vi "Deserialize Object UPDT (XML).vi"(8 "error in":errorcluster, 9 "values":string[](array[string]), 10 "names":string[](array[string]), 11 "object type":refnum<class "_ISerializable.lvclass">) -> (0 "error out":errorcluster, 3 "object out":refnum<class "_ISerializable.lvclass">)   [LabVIEW 2018, in "Serializer.lvclass"]
uses:
  Serializer.lvclass
  _Serializable Base Object/_ISerializable.lvclass
  <vilib>/xml/Close Reference(Node).vi
  <resource>/objmgr/DOMUserDefRef.rc
  <vilib>/xml/NI_XML.lvlib
panel:
  out "XML":string
  out "object xml string":string
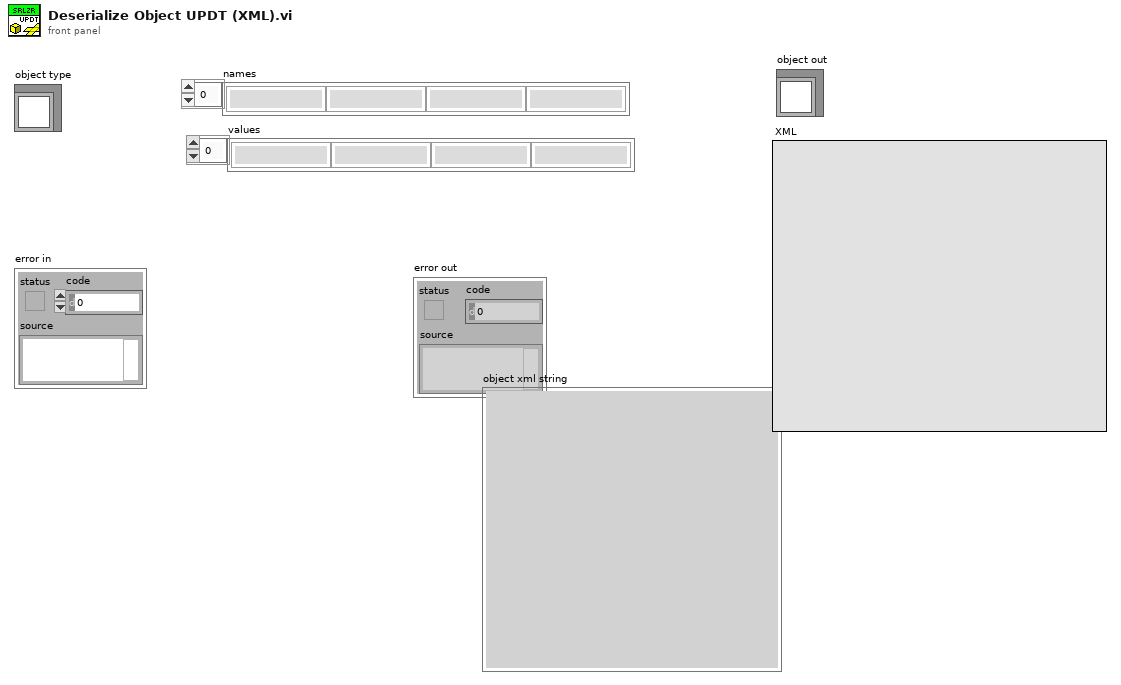
[diagram p1: front panel]
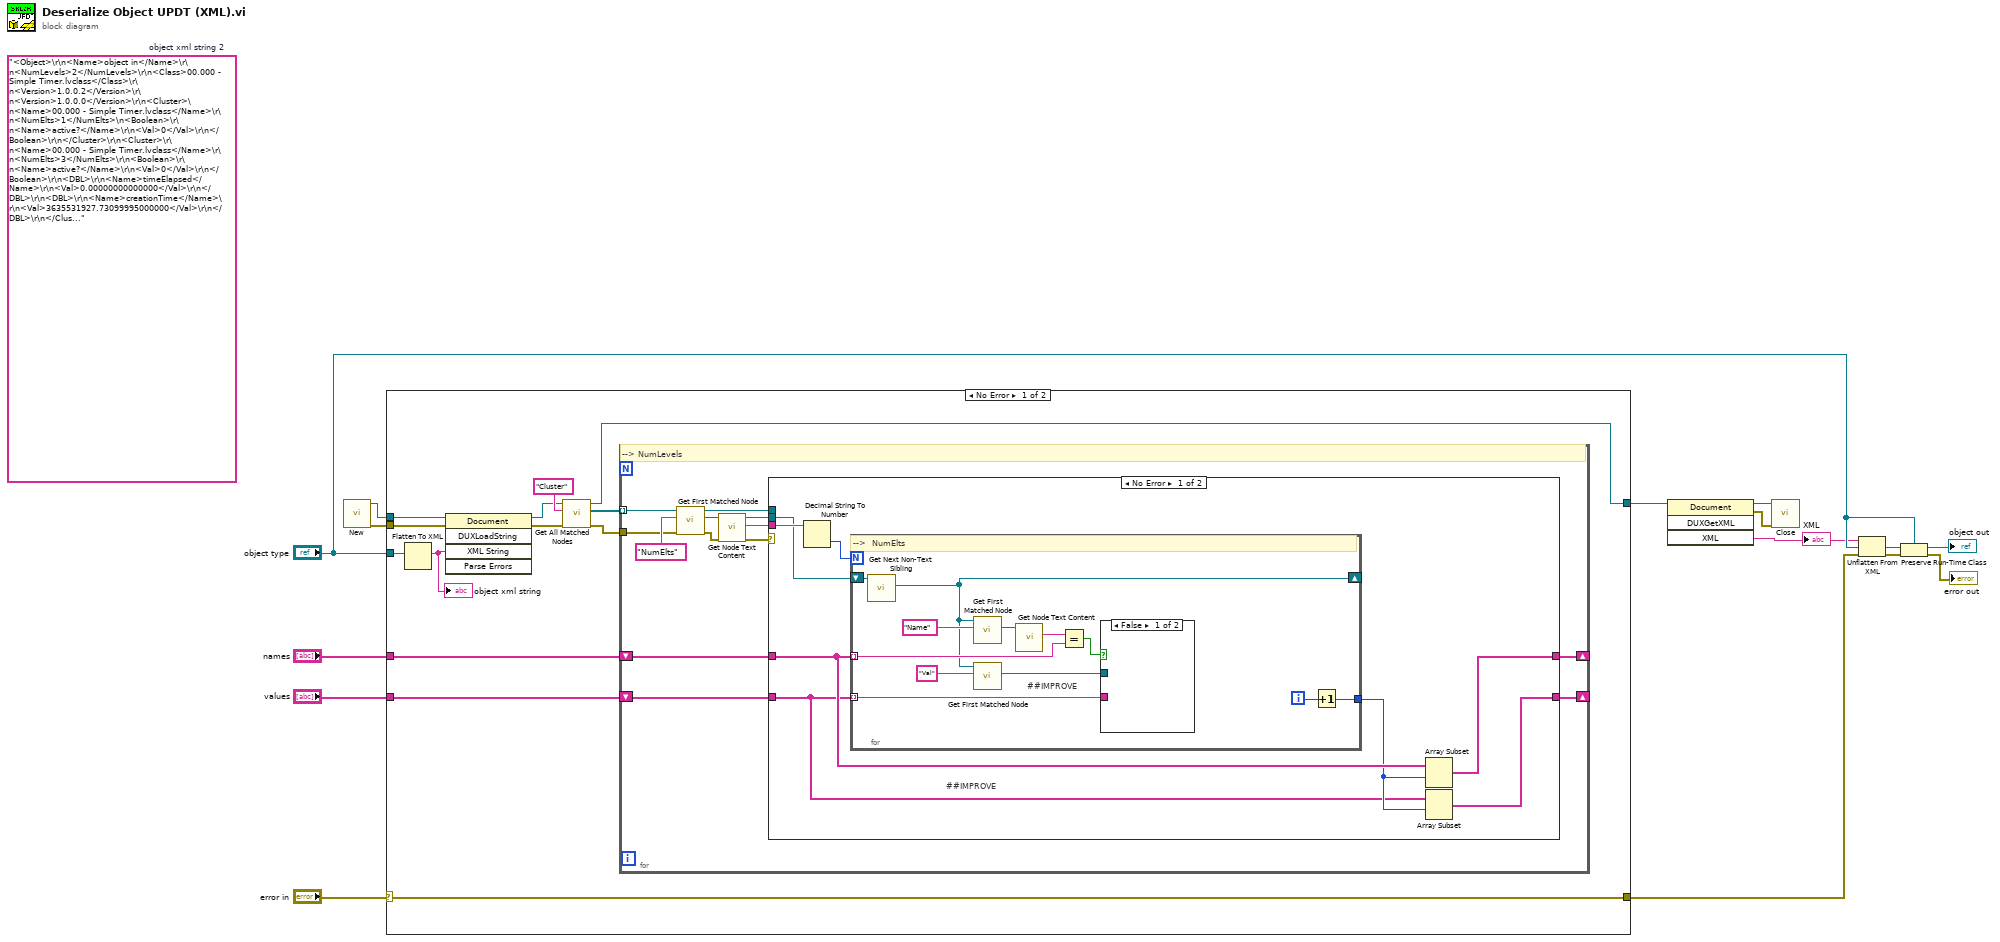
[diagram p0: block diagram]
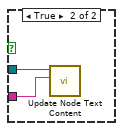
[diagram p2: hidden frame]
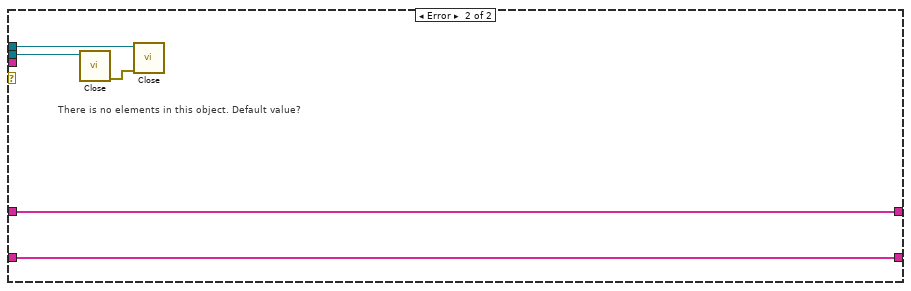
[diagram p3: hidden frame]
diagram:
  (unwired) "<Object>\r\n<Name>object in</Name>\r\n<NumLevels>2</NumLevels>\r\n<Class>00.000 - Simple Timer.lvclass</Class>\r\n<Version>1.0.0.2</Version>\r\n<Version>1.0.0.0</Version>\r\n<Cluster>\n<Name>00.000 - Simple Timer.lvclass</Name>\r\n<NumElts>1</NumElts>\n<Boolean>\r\n<Name>active?</Name>\r\n<Val>0</Val>\r\n</Boolean>\r\n</Cluster>\r\n<Cluster>\r\n<Name>00.000 - Simple Timer.lvclass</Name>\r\n<NumElts>3</NumElts>\r\n<Boolean>\r\n<Name>active?</Name>\r\n<Val>0</Val>\r\n</Boolean>\r\n<DBL>\r\n<Name>timeElapsed</Name>\r\n<Val>0.00000000000000</Val>\r\n</DBL>\r\n<DBL>\r\n<Name>creationTime</Name>\r\n<Val>3635531927.73099995000000</Val>\r\n</DBL>\r\n</Cluster>\r\n</Object>\r\n"  # object xml string 2
  n1 = call <vilib>:"New.vi"() -> ("error out"=w13:errorcluster, "DOM document out"=w12:refnum<k20>)  [unwired: 8 in]
  n2 = case shown="No Error" "error in" {
    selector: "error in" -> [w28 w70]
    tunnel: [w28 w70] -> w4
    tunnel: "object type" -> [w27 _]
    tunnel: w13 -> [w25 _]
    tunnel: w12 -> [w24 w69]
    tunnel: [w21 w69] -> w11
    tunnel: "names" -> [w18 _]
    tunnel: "values" -> [w17 _]
    frame No Error {
      n3 = Flatten To XML(anything=w27) -> (xml string=w16:string)
      "object xml string" <- w16
      n4 = invoke class="Document" method="DUXLoadString"(reference=w24, error in=w25, "XML String"=w16) -> (reference out=w20:refnum<k20>, error out=w23:errorcluster)  [unwired: 2 in, 3 out]
      n5 = call <vilib>:"Get All Matched Nodes.vi"("error in (no error)"=w23, "XPath expression"="Cluster", "node in"=w20) -> ("error out"=w22:errorcluster, "node result array"=w19:refnum<k20>[], "node out"=w21:refnum<k20>)  [unwired: 6 in]
      n6 = for {
        tunnel: w22 -> [w39]
        tunnel: w19 -> [w33] mode=indexing
        shift-right: [w30] -> _
        shift-left: w18 -> [w32]
        shift-right: [w29] -> _
        shift-left: w17 -> [w31]
        # "--> NumLevels"
        n7 = call <vilib>:"Get First Matched Node.vi"("error in (no error)"=w39, "XPath expression"="NumElts", "node in"=w33) -> ("error out"=w35:errorcluster, "node result"=w40:refnum<k20>, "node out"=w36:refnum<k20>)  [unwired: 6 in]
        n8 = call <vilib>:"Get Node Text Content.vi"("error in (no error)"=w35, "node in"=w40) -> ("error out"=w34:errorcluster, "node text"=w38:string, "node out"=w37:refnum<k20>)  [unwired: 7 in]
        n9 = case shown="No Error" w34 {
          tunnel: w38 -> [w49 _]
          tunnel: w37 -> [w47 w68]
          tunnel: w36 -> [_ w67]
          tunnel: w32 -> [w46 w65]
          tunnel: w31 -> [w42 w64]
          tunnel: [w44 w65] -> w30
          tunnel: [w43 w64] -> w29
          frame No Error {
            # "##IMPROVE"
            n10 = Decimal String To Number(string=w49) -> (number=w48:i32)  [unwired: 2 in, 1 out]
            n11 = for {
              N: w48 -> [_]
              shift-right: [w54] -> _
              shift-left: w47 -> [w61]
              tunnel: w46 -> [w56] mode=indexing
              tunnel: w42 -> [w53] mode=indexing
              tunnel: [w50] -> w45
              i -> [w51]
              # "##IMPROVE"
              # "-->  NumElts"
              n12 = call <vilib>:"Get Next Non-Text Sibling.vi"("node in"=w61) -> ("sibling node"=w54:refnum<k20>)  [unwired: 7 in, 3 out]
              n13 = call <vilib>:"Get First Matched Node.vi"("XPath expression"="Name", "node in"=w54) -> ("node result"=w58:refnum<k20>)  [unwired: 7 in, 2 out]
              n14 = call <vilib>:"Get First Matched Node.vi"("XPath expression"="Val", "node in"=w54) -> ("node result"=w55:refnum<k20>)  [unwired: 7 in, 2 out]
              n15 = call <vilib>:"Get Node Text Content.vi"("node in"=w58) -> ("node text"=w57:string)  [unwired: 8 in, 2 out]
              n16 = Equal?(x=w57, y=w56) -> (x = y?=w52:bool)
              n17 = case shown="False" w52 {
                tunnel: w55 -> [_ w63]
                tunnel: w53 -> [_ w62]
                frame False {
                }
                frame True {
                  n18 = call "Update Node Text Content.vi"("node text"=w62, "node in"=w63) -> ()  [unwired: 8 in, 2 out]
                }
              }
              n19 = Increment(x=w51) -> (x+1=w50:i32)
            }
            n20 = Array Subset(array=w46, index=w45) -> (w44:string[])  [unwired: 1 in]
            n21 = Array Subset(array=w42, index=w45) -> (w43:string[])  [unwired: 1 in]
          }
          frame Error {
            # "There is no elements in this object. Default value?"
            n22 = call-poly <vilib>:"Close.vi"("node"=w68) -> ("error out"=w66:errorcluster)  [unwired: 8 in]
            n23 = call-poly <vilib>:"Close.vi"("error in (no error)"=w66, "node"=w67) -> ()  [unwired: 7 in, 1 out]
          }
        }
      }
    }
    frame Error {
    }
  }
  n24 = invoke class="Document" method="DUXGetXML"(reference=w11) -> (reference out=w10:refnum<k20>, error out=w7:errorcluster, "XML"=w8:string)  [unwired: 3 in, 1 out]
  "XML" <- w8
  n25 = call-poly <vilib>:"Close.vi"("error in (no error)"=w7, "node"=w10) -> ()  [unwired: 7 in, 1 out]
  n26 = Unflatten From XML(xml string=w8, type="object type", error in (no error)=w4) -> (value=w6:refnum<class "_ISerializable.lvclass">, error out=w5:errorcluster)
  n27 = Preserve Run-Time Class(object in=w6, error in=w5, 2:"object type") -> (object out=→"object out":refnum<class "_ISerializable.lvclass">, error out=→"error out":errorcluster)
